vi "Serial Test GB_TSFTS2.vi"(8 "error in (no error)":errorcluster) -> (0 "error out":errorcluster, 2 "Message OUT":string, 3 "Result (bool)":bool)   [LabVIEW 2022 SP3]
uses:
  <vilib>/Instr/_visa.llb/VISA Flush IO Buffer Mask.ctl
  <vilib>/Instr/_visa.llb/VISA Configure Serial Port (Instr).vi
panel:
  out "Expected Result":string
  out "Actual Result":string
  out "Result (color)":u32(colorbox)
  out "VISA resource OUT":refnum<visa-resource-name>
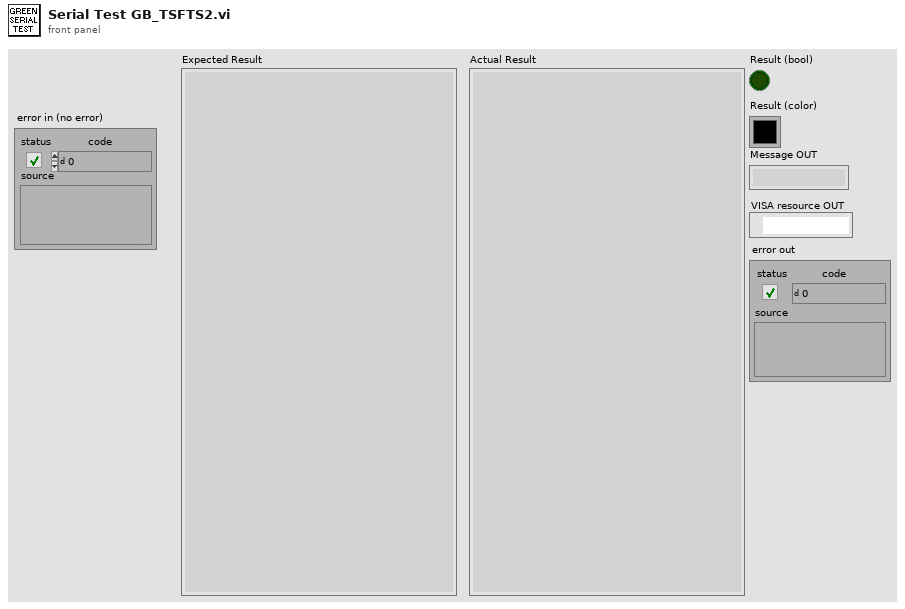
[diagram p1: front panel]
types:
  T1 = typedef "VISA Flush IO Buffer Mask.ctl" = u16
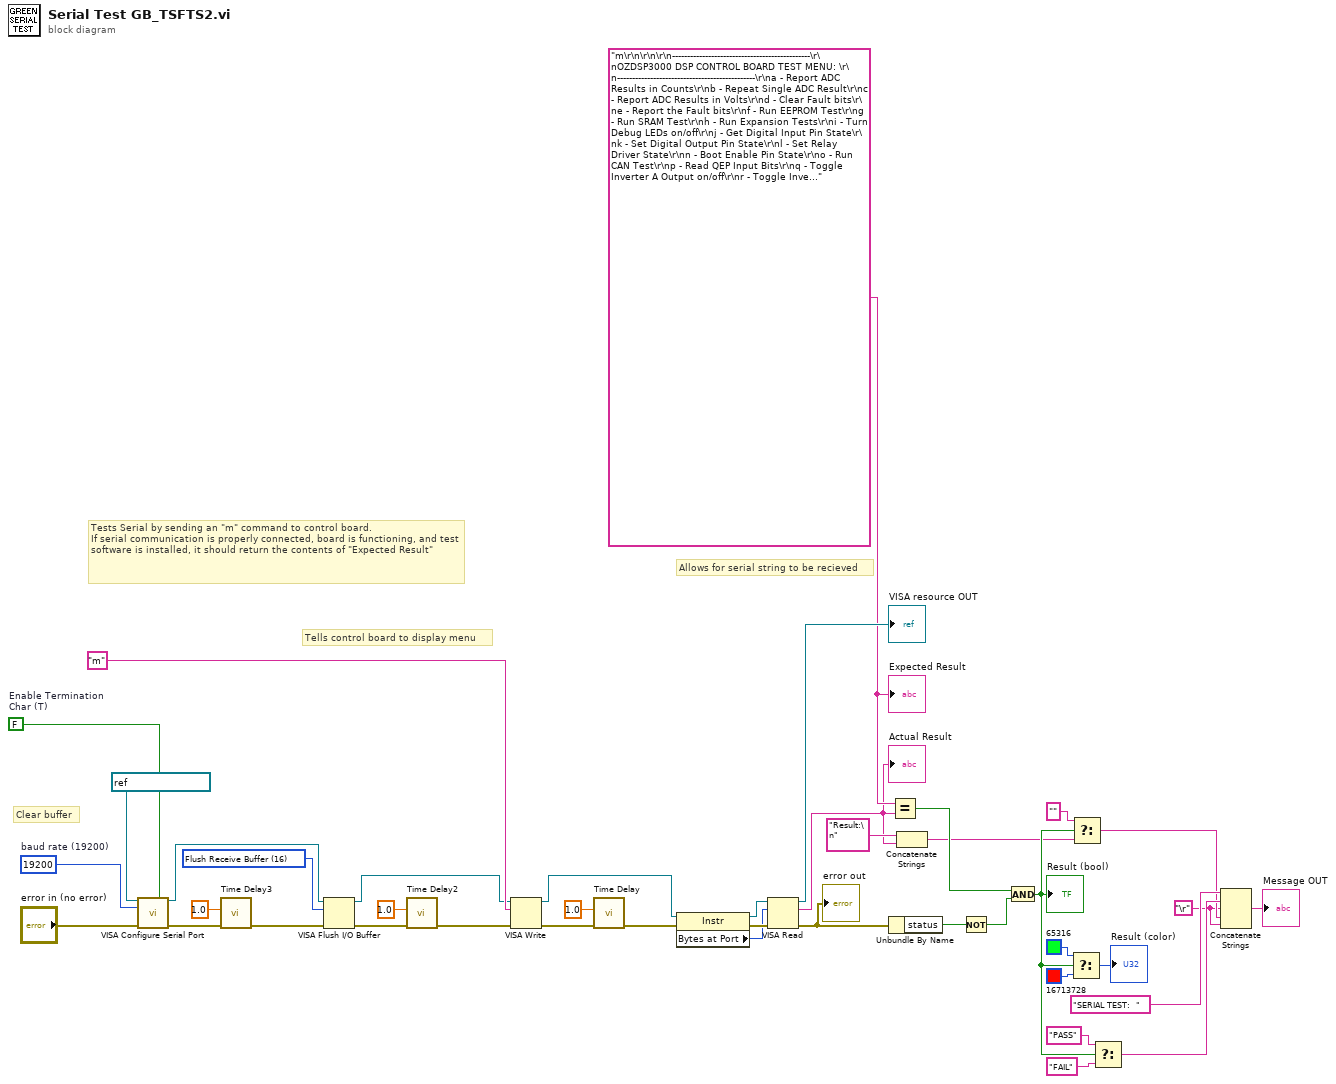
[diagram p0: block diagram]
diagram:
  w9 = "\r"
  w17 = FALSE  # Enable Termination Char (T)
  w18 = u32 19200  # baud rate (19200)
  w23 = "m\r\n\r\n\r\n----------------------------------------------\r\nOZDSP3000 DSP CONTROL BOARD TEST MENU: \r\n----------------------------------------------\r\na - Report ADC Results in Counts\r\nb - Repeat Single ADC Result\r\nc - Report ADC Results in Volts\r\nd - Clear Fault bits\r\ne - Report the Fault bits\r\nf - Run EEPROM Test\r\ng - Run SRAM Test\r\nh - Run Expansion Tests\r\ni - Turn Debug LEDs on/off\r\nj - Get Digital Input Pin State\r\nk - Set Digital Output Pin State\r\nl - Set Relay Driver State\r\nn - Boot Enable Pin State\r\no - Run CAN Test\r\np - Read QEP Input Bits\r\nq - Toggle Inverter A Output on/off\r\nr - Toggle Inverter B Output on/off\r\ns - Toggle Half Bridge Output on/off\r\nt - Set PWM leg duty cycle\r\nu - Real Time Clock\r\nv - Watchdog Control\r\nw - Test Interrupt Lines\r\nx - Read HALLs\r\ny - Test FPGA Read/Write\r\nz - Report Software/FPGA Revs\r\nm - Display this menu\r\n> "
  w38 = T1 16 items=["Flush Receive Buffer"=16, "Write Transmit Buffer to Device"=32, "Flush Receive Buffer (No I/O)"=64, "Flush Transmit Buffer"=128] ("Mask")
  # "Tests Serial by sending an \"m\" command to control board.\nIf serial communication is properly connected, board is functioning, and test software is installed, it should return the contents of \"Expected Result\""
  # "Clear buffer"
  # "Allows for serial string to be recieved"
  # "Tells control board to display menu"
  n1 = call-poly "VISA Configure Serial Port"("VISA resource name"=refnum<visa-resource-name> "ControlBoard" ("ControlBoard VISA"), "Enable Termination\nChar (T)"=w17, "baud rate (9600)"=w18, "error in (no error)"="error in (no error)") -> ("VISA resource name out"=w20:refnum<visa-resource-name>, "error out"=w6:errorcluster)  [unwired: 10 in]
  n2 = call "Time Delay3"("error in (no error)"=w6, "Delay Time (s)"=1.0) -> ("error out"=w5:errorcluster)  [unwired: 9 in]
  n3 = VISA Flush I/O Buffer(VISA resource name=w20, mask (16)=w38, error in (no error)=w5) -> (VISA resource name out=w36:refnum<visa-resource-name>, error out=w8:errorcluster)
  n4 = call "Time Delay2"("error in (no error)"=w8, "Delay Time (s)"=1.0) -> ("error out"=w7:errorcluster)  [unwired: 9 in]
  n5 = VISA Write(VISA resource name=w36, write buffer="m", error in (no error)=w7) -> (VISA resource name out=w34:refnum<visa-resource-name>, error out=w37:errorcluster)  [unwired: 1 out]
  n6 = call "Time Delay"("error in (no error)"=w37, "Delay Time (s)"=1.0) -> ("error out"=w35:errorcluster)  [unwired: 9 in]
  n7 = property class="Instr"(reference=w34, error in=w35) -> (reference out=w41:refnum<visa-resource-name>, error out=w40:errorcluster, "Bytes at Port"=w39:u32)
  n8 = VISA Read(VISA resource name=w41, byte count=w39, error in (no error)=w40) -> (VISA resource name out=→"VISA resource OUT":refnum<visa-resource-name>, read buffer=w14:string, error out=w24:errorcluster)  [unwired: 1 out]
  "error out" <- w24
  "Actual Result" <- w14
  n9 = Unbundle By Name(w24) -> ("status"=w31:bool)
  n10 = Equal?(x=w23, y=w14) -> (x = y?=w25:bool)
  n11 = Concatenate Strings("Result:\n", w14) -> (w11:string)
  n12 = Not(x=w31) -> (.not. x?=w32:bool)
  n13 = And(x=w25, y=w32) -> (x .and. y?=w13:bool)
  "Result (bool)" <- w13
  n14 = Select(t=u32 65316 ("Result (color)"), s=w13, f=u32 16713728 ("Result (color)")) -> (s? t:f=→"Result (color)":u32)
  n15 = Select(t="", s=w13, f=w11) -> (s? t:f=w12:string)
  n16 = Select(t="PASS", s=w13, f="FAIL") -> (s? t:f=w16:string)
  n17 = Concatenate Strings("SERIAL TEST:  ", w16, w9, w12, w9) -> (→"Message OUT":string)
  "Expected Result" <- w23
